vi "Read Rate (Hz).vi"(8 "error in (no error)":errorcluster, 11 "Gate in":refnum<class "Gate.lvclass">) -> (0 "error out":errorcluster, 2 "Rate (Hz)":dbl, 3 "Gate out":refnum<class "Gate.lvclass">)   [LabVIEW 2020, in "Gate.lvclass"]
uses:
  Gate.lvclass
  Gate.lvclass/Gate.ctl
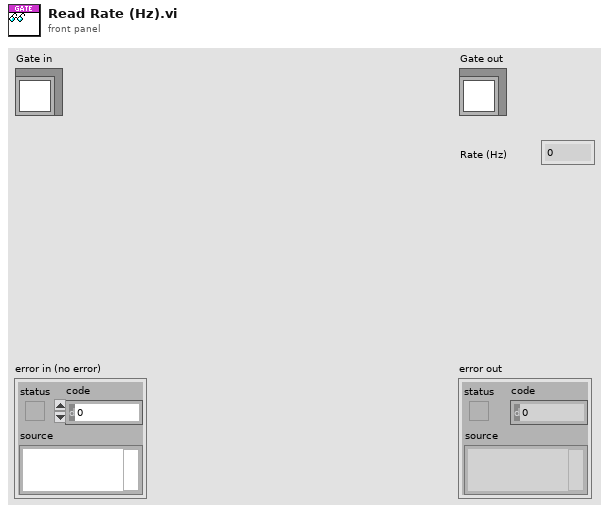
[diagram p1: front panel]
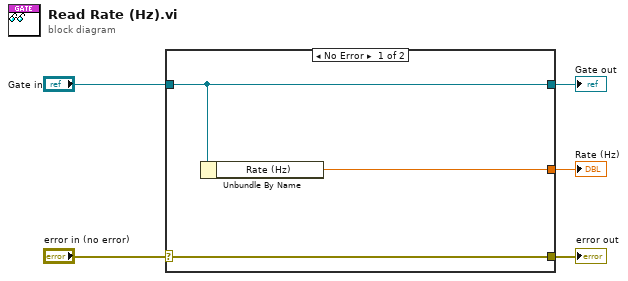
[diagram p0: block diagram]
diagram:
  n1 = case shown="No Error" "error in (no error)" {
    selector: "error in (no error)" -> [w8 w9]
    tunnel: [w8 w9] -> w4
    tunnel: [w7 w10] -> w2
    tunnel: "Gate in" -> [w7 w10]
    tunnel: [w6 _] -> w1
    frame No Error {
      n2 = Unbundle By Name(w7) -> ("Rate (Hz)"=w6:dbl)
    }
    frame Error {
    }
  }
  "error out" <- w4
  "Gate out" <- w2
  "Rate (Hz)" <- w1
